vi "Exemple_Metrics_Brier_Score_Loss.vi"() -> ()   [LabVIEW 2020]
uses:
  Objet/3 - Model selection and evaluation/3.3 - Metrics and scoring/brier_score_loss/Brier_Score_Loss.vi
panel:
  out "Score":string
  out "error out":errorcluster caption="sortie d'erreur"
  in  "error in (no error)":errorcluster caption="entrée d'erreur (pas d'erreur)"
  in  "brier_score_loss":T1={"sample_weight"=[], "pos_label"={"dtype_pos_label"="None", "pos_label"="None"}}
  in  "y_prob":string[][](array[string])=[["0,1"], ["0,9"], ["0,8"], ["0,3"]]
  in  "y_true":string[][](array[string])=[["0"], ["1"], ["1"], ["0"]]
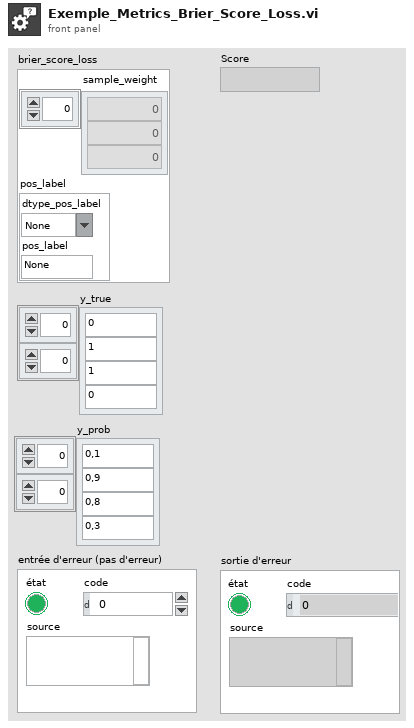
[diagram p1: front panel]
types:
  T1 = cluster{"sample_weight":dbl[], "pos_label":cluster{"dtype_pos_label":string, "pos_label":string}}
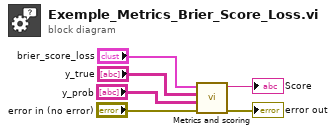
[diagram p0: block diagram]
diagram:
  n1 = call-poly "Metrics and scoring.vi"("error in (no error)"="error in (no error)", "y_prob"="y_prob", "y_true"="y_true", "brier_score_loss"="brier_score_loss") -> ("error out"=→"error out":errorcluster, "Score"=→"Score":string)  [unwired: 6 in]
